vi "getType.vi"(8 "error in (no error)":errorcluster, 11 "tBSONBinary in":refnum<class "tBSONBinary.lvclass">) -> (0 "error out":errorcluster, 2 "Type":T1 items=["unknown"=0, "double"=1, "string"=2, "document"=3, "array"=4, "binary"=5, "objectID"=7, "boolean"=8, "utc datetime"=9, "null"=10, "regular expression"=11, "javascript code"=13, "symbol"=14, "javascript code w/ scope"=15, "i32"=16, "timestamp"=17, "i64"=18, "min key"=255, "max key"=127], 3 "tBSONBinary out":refnum<class "tBSONBinary.lvclass">)   [LabVIEW 2013, in "BSON.lvlib" / "tBSONBinary.lvclass"]
uses:
  tBSONBinary.lvclass
  tBSONElement/type.ctl
  tBSONElement/tBSONElement.lvclass
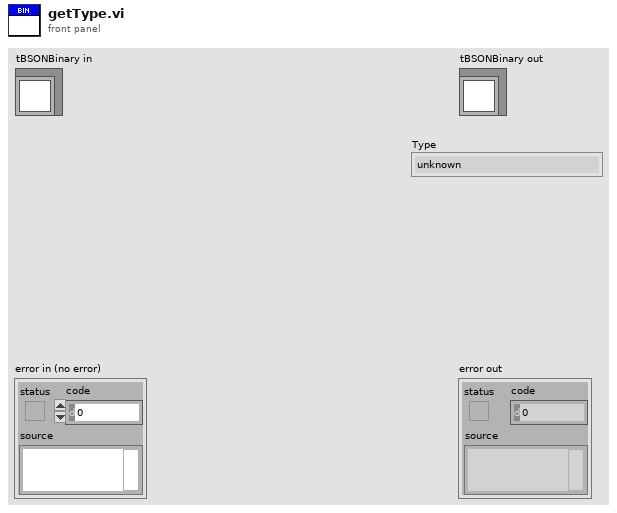
[diagram p1: front panel]
types:
  T1 = typedef "BSON.lvlib/tBSONElement.lvclass/type.ctl" = u8
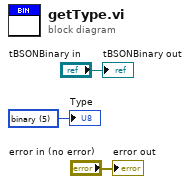
[diagram p0: block diagram]
diagram:
  w3 = T1 5 items=["unknown"=0, "double"=1, "string"=2, "document"=3, "array"=4, "binary"=5, "objectID"=7, "boolean"=8, "utc datetime"=9, "null"=10, "regular expression"=11, "javascript code"=13, "symbol"=14, "javascript code w/ scope"=15, "i32"=16, "timestamp"=17, "i64"=18, "min key"=255, "max key"=127] ("Type")
  "error out" <- "error in (no error)"
  "tBSONBinary out" <- "tBSONBinary in"
  "Type" <- w3
